vi "run.create.from_json.vi"(8 "error in":errorcluster, 10 "JSON":string, 11 "Nominal Client":refnum<class "Nominal Client.lvclass">) -> (0 "error out":errorcluster, 3 "Run out":refnum<class "Run.lvclass">)   [LabVIEW 2020, in "Nominal Client.lvclass"]
uses:
  Nominal Client.lvclass
  Run/Run.lvclass
  Run/Run.lvclass/Run.ctl
  Run/client.set.vi
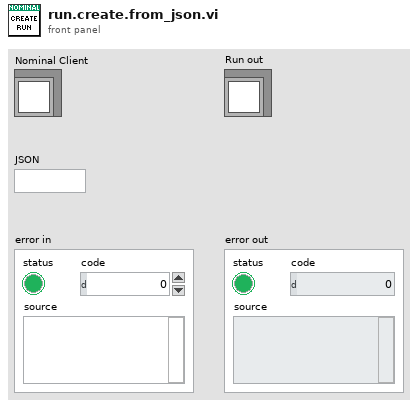
[diagram p1: front panel]
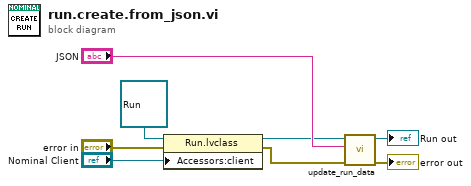
[diagram p0: block diagram]
diagram:
  n1 = property class="Run.lvclass"(reference=refnum<class "Run.lvclass"> refnum ("Run out"), error in="error in", "Accessors:client"="Nominal Client") -> (reference out=w4:refnum<class "Run.lvclass">, error out=w2:errorcluster)
  n2 = call "update_run_data.vi"("error in"=w2, "Run JSON"="JSON", "Run in"=w4) -> ("error out"=→"error out":errorcluster, "Run out"=→"Run out":refnum<class "Run.lvclass">)  [unwired: 7 in]
